vi "Handle Value Change.vi"(5 "VolatusAPI":refnum<class "VolatusAPI.lvclass">, 7 "CtlRef":refnum<vi>, 8 "error in (no error)":errorcluster, 9 "NewVal":variant, 10 "OldVal":variant, 11 "BluelinesRedlines in":refnum<class "BluelinesRedlines.lvclass">) -> (0 "error out":errorcluster, 3 "BluelinesRedlines out":refnum<class "BluelinesRedlines.lvclass">)   [LabVIEW 2020, in "VolatusGUIElements.lvlib" / "BluelinesRedlines.lvclass"]
uses:
  BluelinesRedlines.lvclass
  Volatus/VolatusAPI/VolatusAPI.lvclass
  BluelinesRedlines.lvclass/BluelinesRedlines.ctl
  BLRL Control.ctl
  Value Change Data.ctl
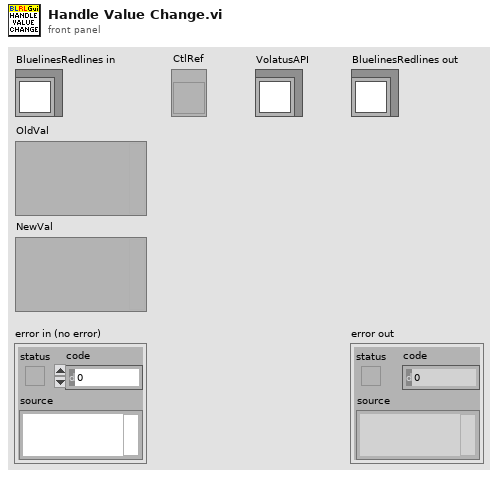
[diagram p1: front panel]
types:
  T1 = typedef "VolatusGUIElements.lvlib/BluelinesRedlines.lvclass/BLRL Control.ctl" = cluster{"Blue Lines":cluster{"Channel":string, "Low":dbl, "Value":dbl, "High":dbl, "Color":u32, "Remove Channel":bool}[], "Red Lines":cluster{"Channel":string, "Low":dbl, "Value":dbl, "High":dbl, "Color":u32, "Remove Channel":bool}[], "Import":bool, "Export":bool, "Blueline Status":bool, "Redlines Status":bool, "Group":string, "New Group":bool, "Dup Group":bool, "Remove Group":bool, "Add Blue Channel":bool, "Add Red Channel":bool}
  T2 = typedef "VolatusGUIElements.lvlib/BluelinesRedlines.lvclass/Value Change Data.ctl" = cluster{"Old":T1, "New":T1}
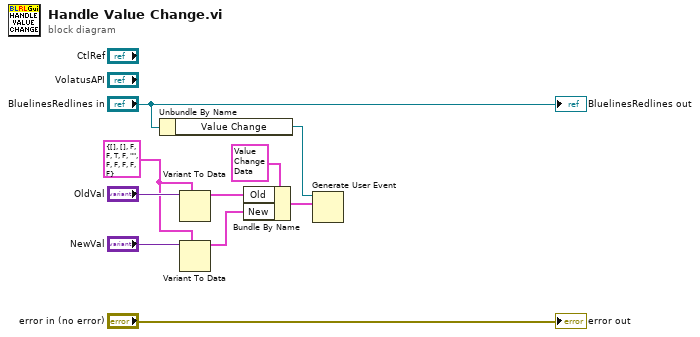
[diagram p0: block diagram]
diagram:
  w3 = T1 {"Blue Lines"=[], "Red Lines"=[], "Import"=FALSE, "Export"=FALSE, "Blueline Status"=TRUE, "Redlines Status"=FALSE, "Group"="", "New Group"=FALSE, "Dup Group"=FALSE, "Remove Group"=FALSE, "Add Blue Channel"=FALSE, "Add Red Channel"=FALSE} ("New")
  n1 = Unbundle By Name("BluelinesRedlines in") -> ("Value Change"=w8:refnum<user-event>)
  n2 = Variant To Data(type=w3, Variant="OldVal") -> (data=w4:T1)  [unwired: 1 in, 1 out]
  n3 = Variant To Data(type=w3, Variant="NewVal") -> (data=w2:T1)  [unwired: 1 in, 1 out]
  n4 = Bundle By Name(cluster=T2 {"Old"={"Blue Lines"=[], "Red Lines"=[], "Import"=FALSE, "Export"=FALSE, "Blueline Status"=FALSE, "Redlines Status"=FALSE, "Group"="", "New Group"=FALSE, "Dup Group"=FALSE, "Remove Group"=FALSE, "Add Blue Channel"=FALSE, "Add Red Channel"=FALSE}, "New"={"Blue Lines"=[], "Red Lines"=[], "Import"=FALSE, "Export"=FALSE, "Blueline Status"=FALSE, "Redlines Status"=FALSE, "Group"="", "New Group"=FALSE, "Dup Group"=FALSE, "Remove Group"=FALSE, "Add Blue Channel"=FALSE, "Add Red Channel"=FALSE}} ("event data"), "Old"=w4, "New"=w2) -> (w6:T2)
  n5 = Generate User Event(user event=w8, event data cluster=w6) -> ()  [unwired: 2 in, 2 out]
  "error out" <- "error in (no error)"
  "BluelinesRedlines out" <- "BluelinesRedlines in"
